vi "读取参数值.vi"(8 "error in (no error)":errorcluster, 10 "Slave ID":u8=1, 11 "MB session in":refnum<class "MB_Master.lvclass">) -> (0 "error out":errorcluster, 1 "Registers":u16[](array[numeric]), 2 "测流参数":T1, 3 "MB session out":refnum<class "MB_Master.lvclass">)   [LabVIEW 2016, in "斯坦道功率测流.lvlib"]
uses:
  <vilib>/Plasmionique/MB Master/MB_Master/MB_Master.lvclass
  <vilib>/Plasmionique/MB Master/MB Master.lvlib
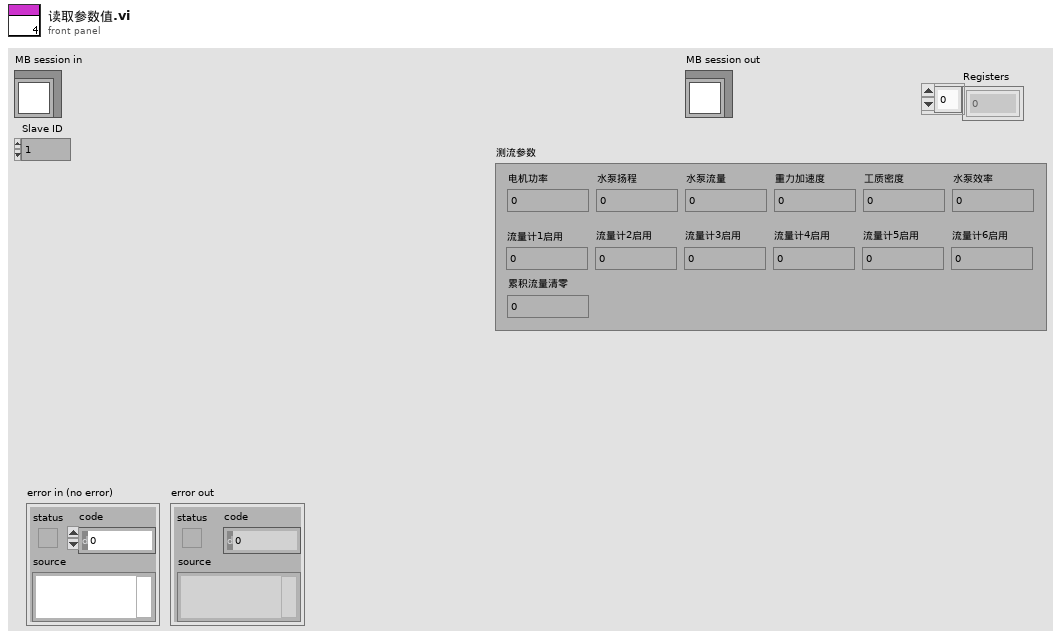
[diagram p1: front panel]
types:
  T1 = typedef "斯坦道功率测流.lvlib/测流参数.ctl" = cluster{"电机功率":dbl, "水泵扬程":dbl, "水泵流量":dbl, "重力加速度":dbl, "工质密度":dbl, "水泵效率":dbl, "流量计1启用":u16, "流量计2启用":u16, "流量计3启用":u16, "流量计4启用":u16, "流量计5启用":u16, "流量计6启用":u16, "累积流量清零":u16}
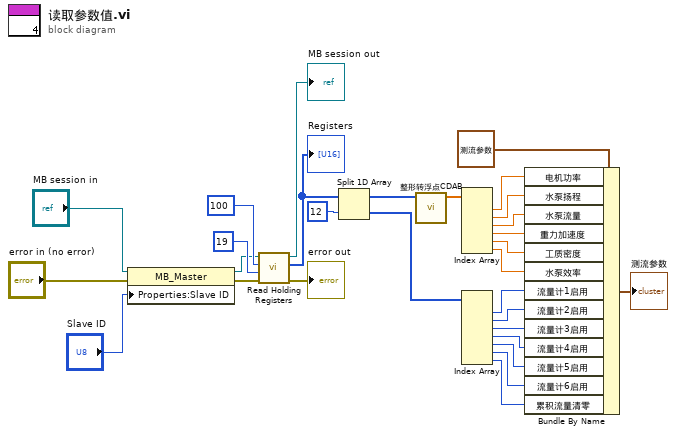
[diagram p0: block diagram]
diagram:
  n1 = property class="MB_Master"(reference="MB session in", error in="error in (no error)", "Properties:Slave ID"="Slave ID") -> (reference out=w24:refnum<class "MB_Master.lvclass">, error out=w22:errorcluster)
  n2 = call <vilib>:"Read Holding Registers.vi"("error in (no error)"=w22, "quantity"=u16 19, "starting address"=u16 100, "MB session in"=w24) -> ("error out"=→"error out":errorcluster, "Registers"=w20:u16[], "MB session out"=→"MB session out":refnum<class "MB_Master.lvclass">)  [unwired: 5 in]
  "Registers" <- w20
  n3 = Split 1D Array(array=w20, index=12 ("索引")) -> (first subarray=w16:u16[], second subarray=w8:u16[])
  n4 = call "整形转浮点CDAB.vi"("数组"=w16) -> ("CDAB"=w15:sgl[])  [unwired: 10 in]
  n5 = Index Array(array=w15) -> (element #1=w14:sgl, element #2=w13:sgl, element #3=w12:sgl, element #4=w11:sgl, element #5=w10:sgl, element #6=w9:sgl)  [unwired: 6 in]
  n6 = Index Array(array=w8) -> (element #1=w7:u16, element #2=w6:u16, element #3=w5:u16, element #4=w4:u16, element #5=w3:u16, element #6=w2:u16, element #7=w1:u16)  [unwired: 7 in]
  n7 = Bundle By Name(cluster=T1 {"电机功率"=0.0, "水泵扬程"=0.0, "水泵流量"=0.0, "重力加速度"=0.0, "工质密度"=0.0, "水泵效率"=0.0, "流量计1启用"=0, "流量计2启用"=0, "流量计3启用"=0, "流量计4启用"=0, "流量计5启用"=0, "流量计6启用"=0, "累积流量清零"=0} ("测流参数"), "电机功率"=w14, "水泵扬程"=w13, "水泵流量"=w12, "重力加速度"=w11, "工质密度"=w10, "水泵效率"=w9, "流量计1启用"=w7, "流量计2启用"=w6, "流量计3启用"=w5, "流量计4启用"=w4, "流量计5启用"=w3, "流量计6启用"=w2, "累积流量清零"=w1) -> (→"测流参数":T1)
